vi "ClearArbWfrm.vi"(8 "error in (no error)":errorcluster, 11 "ClassIn":refnum<class "Keysight335XX.lvclass">) -> (0 "error out":errorcluster, 3 "ClassOut":refnum<class "Keysight335XX.lvclass">)   [LabVIEW 2014, in "FGenPlugins.lvlib" / "Keysight335XX.lvclass"]
uses:
  Keysight335XX.lvclass
  <instrlib>/Agilent 3352X Series/Agilent 3352X Series.lvlib
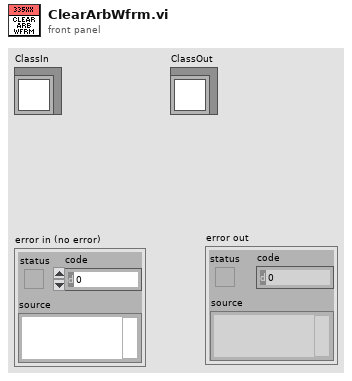
[diagram p1: front panel]
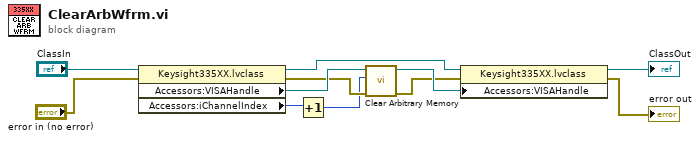
[diagram p0: block diagram]
diagram:
  n1 = property class="Keysight335XX.lvclass"(reference="ClassIn", error in="error in (no error)") -> (reference out=w3:refnum<class "Keysight335XX.lvclass">, error out=w5:errorcluster, "Accessors:VISAHandle"=w7:refnum<visa-resource-name>, "Accessors:iChannelIndex"=w2:i32)
  n2 = Increment(x=w2) -> (x+1=w1:i32)
  n3 = call <instrlib>:"Clear Arbitrary Memory.vi"("error in (no error)"=w5, "Channel (1: 1)"=w1, "VISA resource name"=w7) -> ("error out"=w4:errorcluster, "VISA resource name out"=w6:refnum<visa-resource-name>)  [unwired: 7 in]
  n4 = property class="Keysight335XX.lvclass"(reference=w3, error in=w4, "Accessors:VISAHandle"=w6) -> (reference out=→"ClassOut":refnum<class "Keysight335XX.lvclass">, error out=→"error out":errorcluster)
